vi "Create Configurable SMO Tester.vi"(5 "ConfigManager":refnum<class "ConfigManager.lvclass">, 7 "Config":T1, 8 "error in (no error)":errorcluster, 10 "Subsystem Name (optional)":string, 11 "SMO.Configurable in":refnum<class "SMO.Configurable.lvclass">) -> (0 "error out":errorcluster, 2 "SMO name":string, 3 "SMO.Configurable out":refnum<class "SMO.Configurable.lvclass">)   [LabVIEW 2013, in "SMO.Configurable.lvclass"]
uses:
  SMO.Configurable.lvclass
  Config--cluster.ctl
  <vilib>/LabVIEW Open Source/Configuration Manager/Manager/ConfigManager.lvclass
  src/SMO/SMO.lvclass
  <vilib>/LabVIEW Open Source/Configuration Manager/Cache/ConfigManager.Cache.lvclass
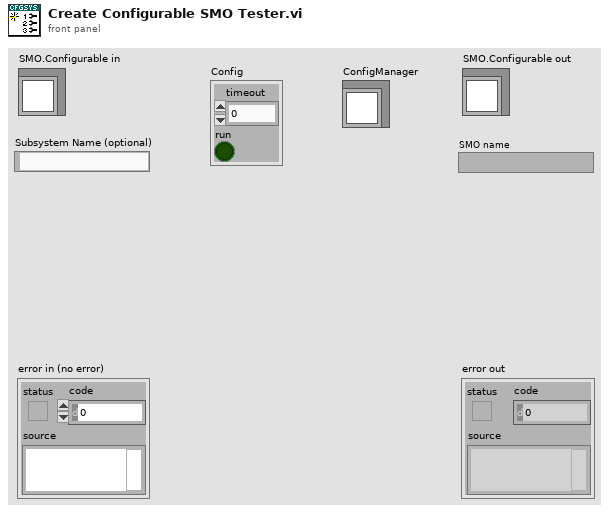
[diagram p1: front panel]
types:
  T1 = typedef "SMO.Configurable.lvclass/Config--cluster.ctl" = cluster{"timeout":i32, "run":bool}
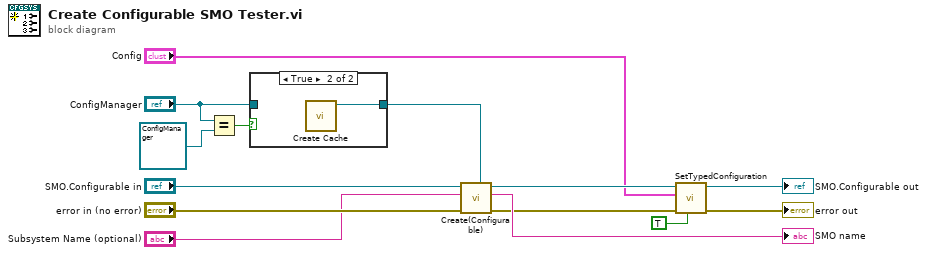
[diagram p0: block diagram]
diagram:
  n1 = Equal?(x="ConfigManager", y=refnum<class "ConfigManager.lvclass"> refnum) -> (x = y?=w3:bool)
  n2 = case shown="True" w3 {
    tunnel: [w15 w16] -> w10
    tunnel: "ConfigManager" -> [w15 _]
    frame False {
    }
    frame True {
      n3 = call <vilib>:"Create Cache.vi"() -> ("ConfigManager.Cache"=w16:refnum<class "ConfigManager.Cache.lvclass">)  [unwired: 11 in]
    }
  }
  n4 = call "Create(Configurable).vi"("ConfigManager"=w10, "error in (no error)"="error in (no error)", "Subsystem Name (optional)"="Subsystem Name (optional)", "SMO"="SMO.Configurable in") -> ("error out"=w9:errorcluster, "SMO name"=→"SMO name":string, "SMO out"=w8:refnum<class "SMO.Configurable.lvclass">)  [unwired: 5 in]
  n5 = call "SetTypedConfiguration.vi"("private? (F)"=TRUE, "error in (no error)"=w9, "Default value"="Config", "SMO"=w8) -> ("error out"=→"error out":errorcluster, "SMO out"=→"SMO.Configurable out":refnum<class "SMO.Configurable.lvclass">)  [unwired: 6 in]
